vi "Sandbox.vi"() -> ()   [LabVIEW 2019]
uses:
  <vilib>/NI VeriStand/VeriStand Data/Pointer Operations/Pointer.Write (1D U8).vi
  <vilib>/NI VeriStand/VeriStand Data/VeriStand Data.lvlib
  <vilib>/NI VeriStand/VeriStand Data/Pointer Operations/Pointer.Read (1D U8).vi
panel:
  in  "count":i32
  out "error out":errorcluster
  out "values":u8[](array[numeric]) format="%02x"
  out "Cast U64 Pointer":u64 format="%016x"
  out "Converted U64 Pointer":u64 format="%016x"
  out "Cast Double Pointer":dbl
  out "Converted Double Pointer":dbl
  out "Original Pointer":u64 format="%016x"
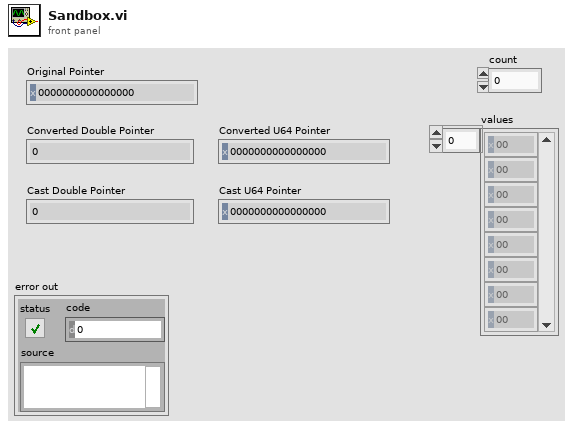
[diagram p1: front panel]
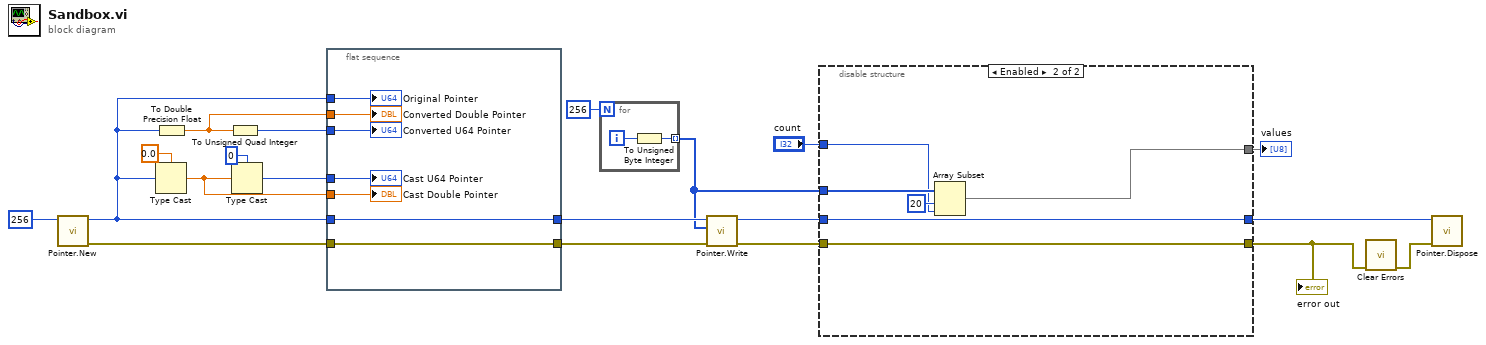
[diagram p0: block diagram]
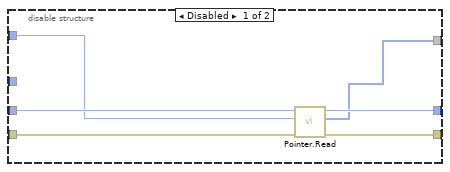
[diagram p2: hidden frame]
diagram:
  n1 = call <vilib>:"Pointer.New.vi"("size in bytes"=u64 256) -> ("error out"=w20:errorcluster, "pointer"=w12:u64)  [unwired: 9 in]
  n2 = Type Cast(type=0.0, x=w12) -> (*(type *) &x=w16:dbl)
  n3 = To Double Precision Float(number=w12) -> (double precision float=w18:dbl)
  n4 = To Unsigned Quad Integer(1:w18) -> (0:w17:u64)
  n5 = Type Cast(type=u64 0, x=w16) -> (*(type *) &x=w13:u64)
  n6 = flat-sequence {
    tunnel: w20 -> [w21]
    tunnel: w18 -> [w27]
    tunnel: w17 -> [w24]
    tunnel: w12 -> [w22]
    tunnel: w16 -> [w26]
    tunnel: w13 -> [w23]
    tunnel: w12 -> [w25]
    tunnel: [w22] -> w11
    tunnel: [w21] -> w10
    frame #0 {
      "Original Pointer" <- w25
      "Converted Double Pointer" <- w27
      "Cast Double Pointer" <- w26
      "Converted U64 Pointer" <- w24
      "Cast U64 Pointer" <- w23
    }
  }
  n7 = for {
    N: 256 -> [_]
    tunnel: [w28] -> w3 mode=indexing
    i -> [w29]
    n8 = To Unsigned Byte Integer(number=w29) -> (unsigned 8bit integer=w28:u8)
  }
  n9 = call-poly <vilib>:"Pointer.Write.vi"("error in (no error)"=w10, "values"=w3, "pointer in"=w11) -> ("error out"=w7:errorcluster, "pointer out"=w8:u64)  [unwired: 6 in, 1 out]
  n10 = disable-structure shown="Enabled" {
    disable-tunnel: w8 -> [w35 w41]
    disable-tunnel: w7 -> [w34 w40]
    disable-tunnel: [w33 w40] -> w6
    disable-tunnel: [w32 w41] -> w4
    disable-tunnel: w3 -> [_ w38]
    disable-tunnel: "count" -> [w31 w37]
    disable-tunnel: [w30 w36] -> w1
    frame Disabled {
      n11 = call-poly <vilib>:"Pointer.Read.vi"("error in (no error)"=w34, "count"=w31, "pointer in"=w35) -> ("error out"=w33:errorcluster, "values"=w30:u8[], "pointer out"=w32:u64)  [unwired: 6 in]
    }
    frame Enabled {
      n12 = Array Subset(array=w38, index=20, length=w37) -> (w36:u8[])
    }
  }
  "error out" <- w6
  "values" <- w1
  n13 = call <vilib>:"Clear Errors.vi"("error in (no error)"=w6) -> ("error out"=w5:errorcluster)  [unwired: 5 in, 1 out]
  n14 = call <vilib>:"Pointer.Dispose.vi"("error in (no error)"=w5, "pointer"=w4) -> ()  [unwired: 8 in, 2 out]
